vi "Configure Output Filter.vi"(6 "Enable Output Filter (T: Enable)":bool=TRUE, 7 "Auto Output Filter (F: Disable)":bool, 8 "error in (no error)":errorcluster, 9 "Cutoff Frequency (31.83)":dbl=31.83, 10 "Channel (0: Channel 1)":i32(ring) items=["Channel 1", "Channel 2"], 11 "VISA resource name":refnum<visa-resource-name>) -> (0 "error out":errorcluster, 3 "VISA resource name out":refnum<visa-resource-name>)   [LabVIEW 2023, in "Agilent B2900 Series.lvlib"]
doc: "Configures the output filter function."
uses:
  Agilent B2900 Series.lvlib
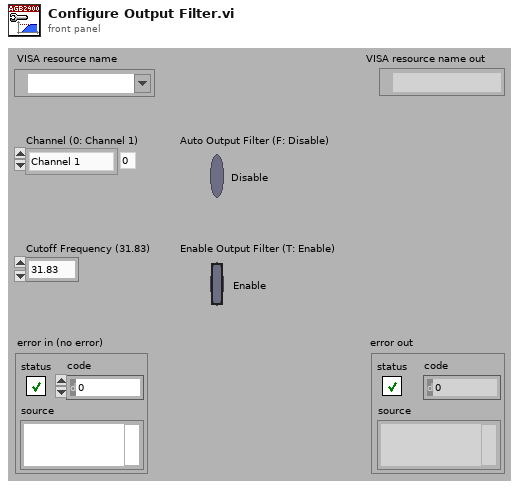
[diagram p1: front panel]
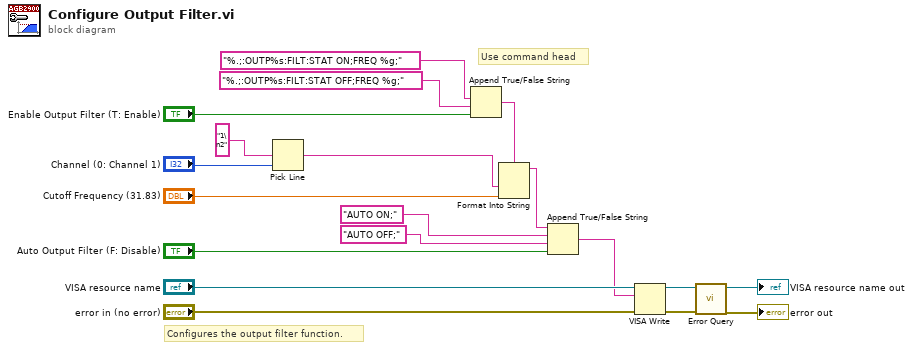
[diagram p0: block diagram]
diagram:
  # "Configures the output filter function."
  # "Use command head"
  n1 = Pick Line(multi-line string="1\n2" ("string (\"\")"), line index="Channel (0: Channel 1)") -> (output string=w4:string)  [unwired: 1 in]
  n2 = Append True/False String(1:"Enable Output Filter (T: Enable)", 2:"%.;:OUTP%s:FILT:STAT OFF;FREQ %g;", 3:"%.;:OUTP%s:FILT:STAT ON;FREQ %g;") -> (0:w6:string)  [unwired: 1 in]
  n3 = Format Into String(format string=w6, w4, "Cutoff Frequency (31.83)") -> (resulting string=w3:string)  [unwired: 2 in, 1 out]
  n4 = Append True/False String(1:"Auto Output Filter (F: Disable)", 2:"AUTO OFF;", 3:"AUTO ON;", 4:w3) -> (0:w1:string)
  n5 = VISA Write(VISA resource name="VISA resource name", write buffer=w1, error in (no error)="error in (no error)") -> (VISA resource name out=w17:refnum<visa-resource-name>, error out=w16:errorcluster)  [unwired: 1 out]
  n6 = call "Error Query.vi"("error in (no error)"=w16, "VISA resource name"=w17) -> ("error out"=→"error out":errorcluster, "VISA resource name out"=→"VISA resource name out":refnum<visa-resource-name>)  [unwired: 6 in, 2 out]
